vi "Cleanup.vi"(8 "error in":errorcluster, 11 "Consolidated_CD in":refnum<class "NIVS_CDEW_MetaDataObj.lvclass">) -> (0 "error out":errorcluster, 3 "Consolidated_CD out":refnum<class "NIVS_CDEW_MetaDataObj.lvclass">)   [LabVIEW 2026, in "NIVS_CDEW_MetaDataObj.lvclass"]
uses:
  NIVS_CDEW_MetaDataObj.lvclass
  NIVS_CDEW_MetaDataObj.lvclass/NIVS_CDEW_MetaDataObj.ctl
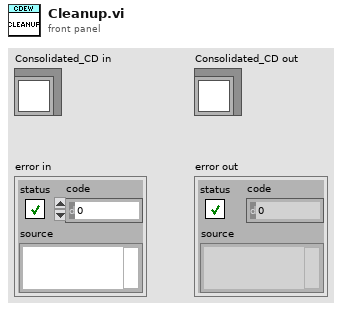
[diagram p1: front panel]
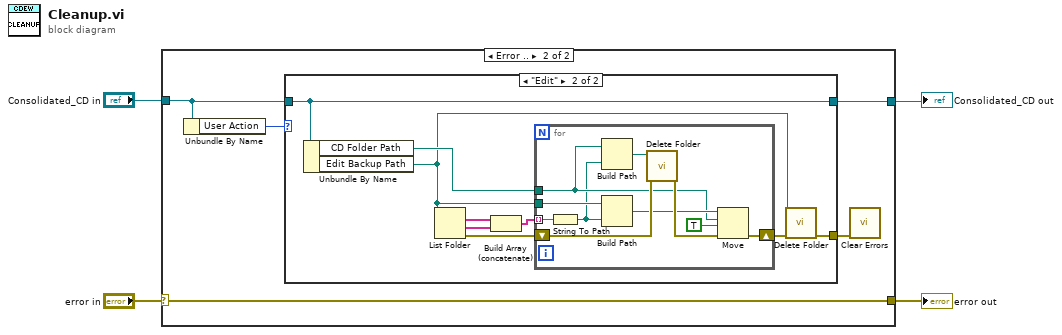
[diagram p0: block diagram]
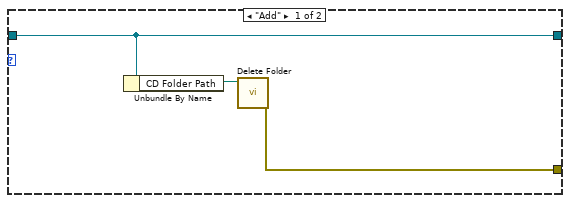
[diagram p3: hidden frame]
diagram:
  n1 = case shown="Error .." "error in" {
    selector: "error in" -> [w6 w11]
    tunnel: [w5 w9] -> w2
    tunnel: "Consolidated_CD in" -> [w5 w8]
    tunnel: [w6 w11] -> w4
    frame No Error {
    }
    frame Error {
      n2 = Unbundle By Name(w8) -> ("User Action"=w7:enum16{"Add", "Edit"})
      n3 = case shown="\"Edit\"" w7 {
        tunnel: [w13 w20] -> w9
        tunnel: w8 -> [w13 w20]
        tunnel: [w14 w21] -> w10
        frame "Add" {
          n4 = Unbundle By Name(w13) -> ("CD Folder Path"=w12:path)
          n5 = call "Delete Folder.vi"("Folder Path"=w12) -> ("error out"=w14:errorcluster)  [unwired: 9 in, 1 out]
        }
        frame "Edit" {
          n6 = Unbundle By Name(w20) -> ("CD Folder Path"=w16:path, "Edit Backup Path"=w15:path)
          n7 = List Folder(path=w15) -> (filenames=w19:string[], folder names=w18:string[], error out=w23:errorcluster)  [unwired: 3 in, 1 out]
          n8 = Build Array (concatenate)(w19, w18) -> (w17:string[])
          n9 = for {
            tunnel: w15 -> [w30]
            tunnel: w17 -> [w29] mode=indexing
            tunnel: w16 -> [w26]
            shift-right: [w33] -> w22
            shift-left: w23 -> [w32]
            n10 = String To Path(string=w29) -> (path=w25:path)
            n11 = Build Path(base path=w26, name or relative path=w25) -> (appended path=w24:path)
            n12 = Build Path(base path=w30, name or relative path=w25) -> (appended path=w28:path)
            n13 = call "Delete Folder.vi"("error in"=w32, "Folder Path"=w24) -> ("error out"=w31:errorcluster)  [unwired: 8 in, 1 out]
            n14 = Move(source path=w28, error in=w31, 9:TRUE ("overwrite (F)"), 10:w26) -> (error out=w33:errorcluster)  [unwired: 1 in, 2 out]
          }
          n15 = call "Delete Folder.vi"("error in"=w22, "Folder Path"=w15) -> ("error out"=w21:errorcluster)  [unwired: 8 in, 1 out]
        }
      }
      n16 = call <vilib>:"Clear Errors.vi"("error in (no error)"=w10) -> ()  [unwired: 5 in, 2 out]
    }
  }
  "error out" <- w4
  "Consolidated_CD out" <- w2
